vi "_InBlacklist.vi"(11 "String":string) -> (3 "in blacklist?":bool)   [LabVIEW 2017, in "RefManager(dev).lvlib"]
uses:
  RefManager(dev).lvlib
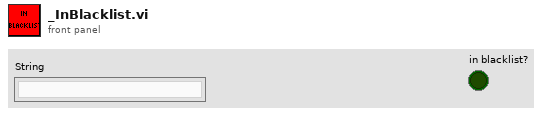
[diagram p1: front panel]
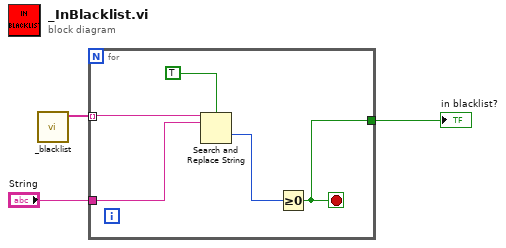
[diagram p0: block diagram]
diagram:
  n1 = call "_blacklist.vi"() -> ("blacklist"=w3:string[])  [unwired: 11 in]
  n2 = for {
    tunnel: w3 -> [w8] mode=indexing
    tunnel: "String" -> [w7]
    tunnel: [w5] -> w1
    stop <- w5 stop-if-true
    n3 = Search and Replace String(case sensitive?=TRUE ("ignore case? (F)"), input string=w8, search string=w7) -> (offset past replacement=w6:i32)  [unwired: 5 in, 3 out]
    n4 = Greater Or Equal To 0?(x=w6) -> (x >= 0?=w5:bool)
  }
  "in blacklist?" <- w1
